vi "U3 2-PWM piezo.vi"(9 "Timer1 Duty Cycle [%]":dbl=50.0 format="%.1f", 10 "8-bit PWM Frequency [Hz]":dbl=40.0 format="%.2f") -> (2 "Actual 8-bit Frequency":dbl format="%.1f")   [LabVIEW 2014]
panel:
  in  "Timer/Counter Pin Offset":u8=4
  out "Update":bool
  out "Timer Value Array":u16[](array[numeric])
  in  "stop":bool
  in  "FirstFound":bool=TRUE
  in  "Address":string="1"
  out "TimerClockDivisor":u8
  out "Error Message":string
  # "Demonstrates 1 channel of 16-bit PWM output and 1 channel of 8-bit PWM output.\nUses the 48 MHz divisor capable clock, and chooses a timer clock divisor to get\nas close as possible to the desired 16-bit PWM frequency.  Since a divisor capable\nclock is used, Counter0 is not available.  Since all timers use the same clock, the\nfrequency of the 8-bit PWM is fixed at 256 times the frequency of the 16-bit PWM.\nIf pin offset is 4, we get:\n\nFIO4 = PWM16\nFIO5 = PWM8"
  # "Range is 2.86 to 732.42 Hz"
  # "This example allows the duty cycles to\nbe changed while the VI is running."
  # "This VI passes a timer\nbase clock constant that\nis valid for hardware V1.21.\nFor hardware V1.20 change\nLJ_tc48MHZ_DIV to LJ_tc24MHZ_DIV."
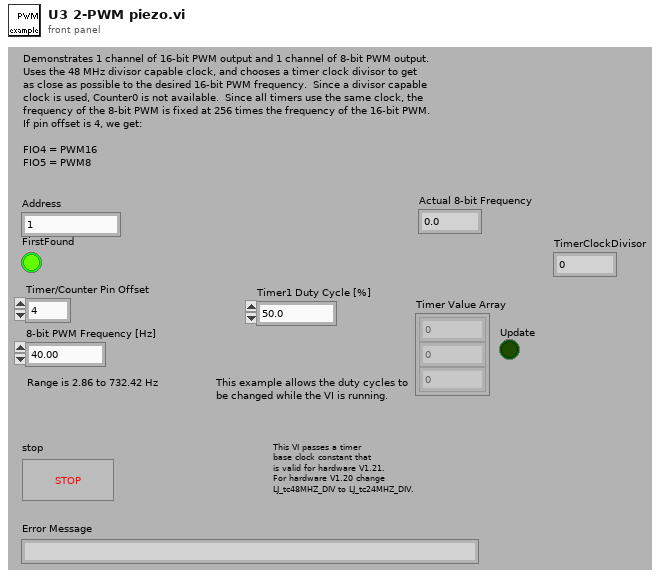
[diagram p1: front panel]
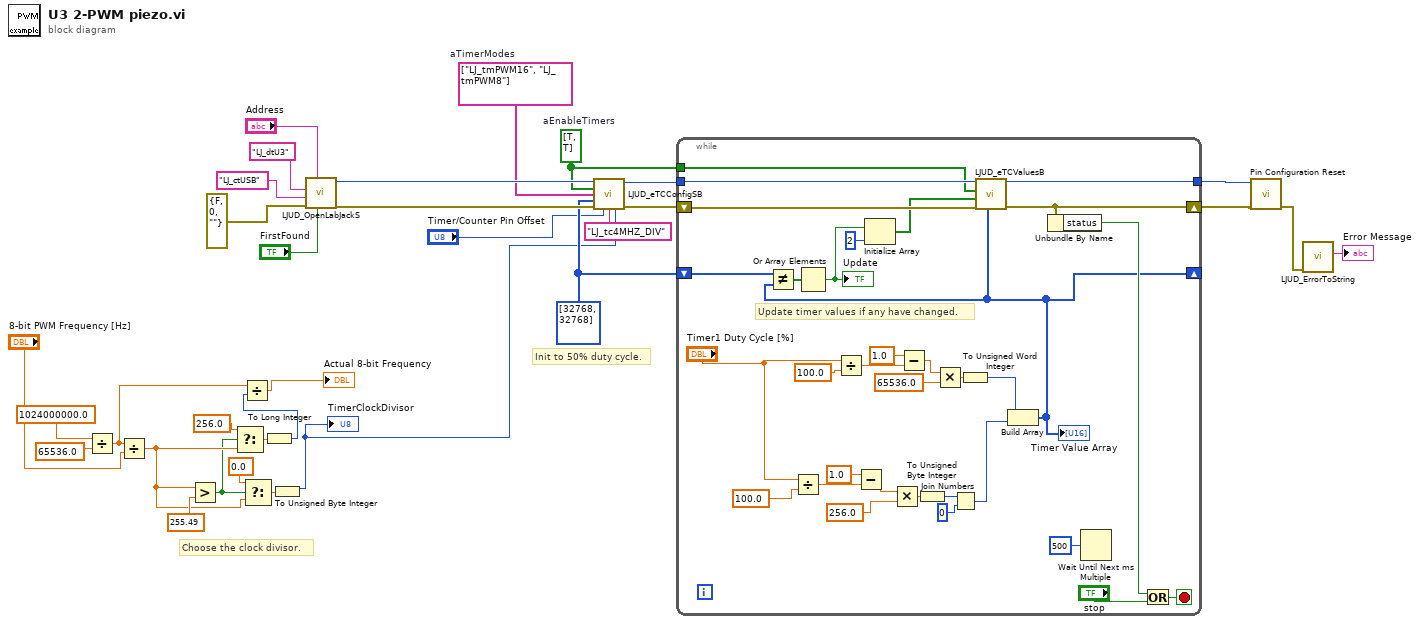
[diagram p0: block diagram]
diagram:
  w2 = bool[] [TRUE, TRUE]  # aEnableTimers
  w7 = string[] ["LJ_tmPWM16", "LJ_tmPWM8"]  # aTimerModes
  w6 = u16[] [32768, 32768] ("TimerValues")
  # "Choose the clock divisor."
  # "Init to 50% duty cycle."
  n1 = Divide(x=1024000000.0, y=65536.0) -> (x/y=w20:dbl)
  n2 = Divide(x=w20, y="8-bit PWM Frequency [Hz]") -> (x/y=w24:dbl)
  n3 = Greater?(x=w24, y=255.49) -> (0:w23:bool)
  n4 = Select(t=256.0, s=w23, f=w24) -> (s? t:f=w26:dbl)
  n5 = Select(t=0.0, s=w23, f=w24) -> (s? t:f=w29:dbl)
  n6 = To Long Integer(number=w26) -> (32bit integer=w22:i32)
  n7 = Divide(x=w20, y=w22) -> (x/y=→"Actual 8-bit Frequency":dbl)
  n8 = To Unsigned Byte Integer(number=w29) -> (unsigned 8bit integer=w3:u8)
  "TimerClockDivisor" <- w3
  n9 = call "LJUD_OpenLabJackS.vi"("FirstFound"="FirstFound", "Address"="Address", "error in"=errorcluster {"status"=FALSE, "code"=0, "source"=""}, "ConnectionType"="LJ_ctUSB", "DeviceType"="LJ_dtU3") -> ("error out"=w8:errorcluster, "Handle"=w9:i32)  [unwired: 4 in, 1 out]
  n10 = call "LJUD_eTCConfigSB.vi"("Handle In"=w9, "aEnableTimers"=w2, "aTimerModes"=w7, "aTimerValues"=w6, "error in"=w8, "TCPinOffset"="Timer/Counter Pin Offset", "TimerClockBase"="LJ_tc4MHZ_DIV" ("Timer Clock Base"), "TimerClockDivisor"=w3) -> ("Handle Out"=w10:i32, "error out"=w11:errorcluster)  [unwired: 6 in]
  n11 = while {
    tunnel: w2 -> [w40]
    tunnel: [w45] -> w18
    shift-left: w6 -> [w52]
    shift-right: [w38] -> _
    tunnel: w10 -> [w42]
    shift-left: w11 -> [w43]
    shift-right: [w44] -> w17
    stop <- w53 stop-if-true
    # "Update timer values if any have changed."
    n12 = Divide(x="Timer1 Duty Cycle [%]", y=100.0) -> (x/y=w64:dbl)
    n13 = Divide(x="Timer1 Duty Cycle [%]", y=100.0) -> (x/y=w58:dbl)
    n14 = Subtract(x=1.0, y=w64) -> (x-y=w36:dbl)
    n15 = Multiply(x=w36, y=256.0) -> (x*y=w61:dbl)
    n16 = Subtract(x=1.0, y=w58) -> (x-y=w56:dbl)
    n17 = To Unsigned Byte Integer(number=w61) -> (unsigned 8bit integer=w37:u8)
    n18 = Multiply(x=w56, y=65536.0) -> (x*y=w55:dbl)
    n19 = Join Numbers(hi=w37, lo=u8 0) -> ((hi.lo)=w46:u16)
    n20 = To Unsigned Word Integer(number=w55) -> (unsigned 16bit integer=w54:u16)
    n21 = Build Array(w54, w46) -> (w38:u16[])
    "Timer Value Array" <- w38
    n22 = Not Equal?(x=w52, y=w38) -> (x != y?=w51:bool[])
    n23 = Or Array Elements(Boolean array=w51) -> (logical OR=w50:bool)
    "Update" <- w50
    n24 = Initialize Array(w50, 2 ("Dimension Size")) -> (w41:bool[])
    n25 = call "LJUD_eTCValuesB.vi"("aTimerValues Write"=w38, "error in"=w43, "aUpdateResetTimers"=w41, "aReadTimers"=w40, "Handle In"=w42) -> ("error out"=w44:errorcluster, "Handle Out"=w45:i32)  [unwired: 3 in, 2 out]
    n26 = Unbundle By Name(w44) -> ("status"=w49:bool)
    n27 = Wait Until Next ms Multiple(millisecond multiple=u32 500) -> ()  [unwired: 1 out]
    n28 = Or(x=w49, y="stop") -> (x .or. y?=w53:bool)
  }
  n29 = call "Pin Configuration Reset.vi"("error in"=w17, "Handle In"=w18) -> ("error out"=w16:errorcluster)  [unwired: 8 in, 1 out]
  n30 = call "LJUD_ErrorToString.vi"("error in"=w16) -> ("String"=→"Error Message":string)  [unwired: 10 in]
